vi "execution class name.vi"(8 "error in":errorcluster, 11 "Tag Bus Web Interface configuration in":refnum<class "Tag Bus Web Interface configuration.lvclass">) -> (0 "error out":errorcluster, 2 "class name":string, 3 "Tag Bus Web Interface configuration out":refnum<class "Tag Bus Web Interface configuration.lvclass">)   [LabVIEW 2013, in "Tag Bus Web Interface configuration.lvclass"]
doc: "Provides an interface for determining the module runtime class associated with this module configuration. This class name can then be used to dynamically load or locate the runtime class for initialization purposes."
uses:
  Tag Bus Web Interface configuration.lvclass
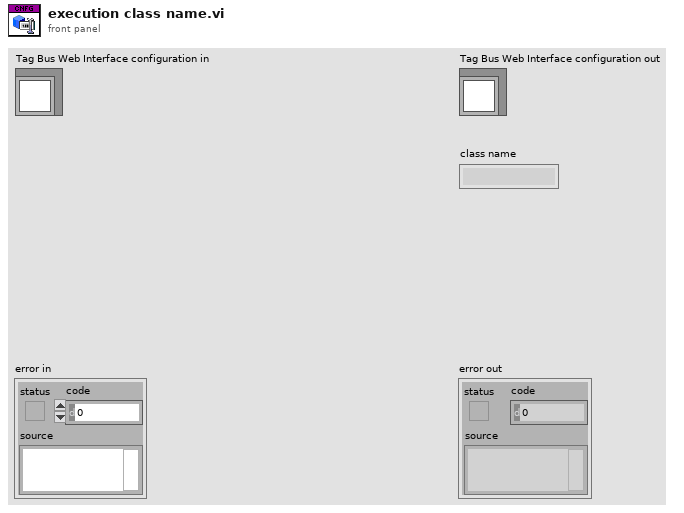
[diagram p1: front panel]
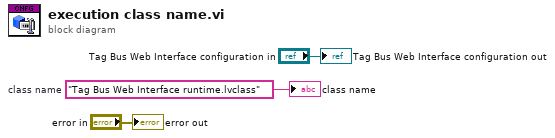
[diagram p0: block diagram]
diagram:
  w1 = "Tag Bus Web Interface runtime.lvclass"  # class name
  "error out" <- "error in"
  "Tag Bus Web Interface configuration out" <- "Tag Bus Web Interface configuration in"
  "class name" <- w1
